vi "Close.vi"(8 "error in (no error)":errorcluster, 11 "ProPar in":refnum<class "PL Bronkhorst ProPar.lvclass">) -> (0 "error out":errorcluster)   [LabVIEW 2015, in "PL Bronkhorst ProPar.lvclass"]
doc: "Closes connection to device."
uses:
  PL Bronkhorst ProPar.lvclass
  PL Bronkhorst ProPar.lvclass/PL Bronkhorst ProPar.ctl
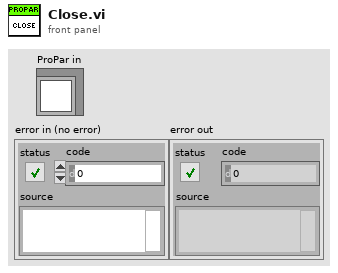
[diagram p1: front panel]
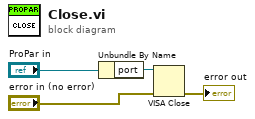
[diagram p0: block diagram]
diagram:
  n1 = Unbundle By Name("ProPar in") -> ("port"=w3:refnum<visa-resource-name>)
  n2 = VISA Close(VISA resource name=w3, error in (no error)="error in (no error)") -> (error out=→"error out":errorcluster)
